vi "my trafic light control.vi"() -> ()   [LabVIEW 2018]
panel:
  in  "stop":bool
  in  "START":bool
  out "Timer 4":u8
  out "Timer 3":u8
  out "Timer 2":u8
  out "Timer":u8
  out "Traffic Light 4":cluster{"Red":bool, "Yellow":bool, "Green":bool}
  out "Traffic Light 3":cluster{"Red":bool, "Yellow":bool, "Green":bool}
  out "Traffic Light 2":cluster{"Red":bool, "Yellow":bool, "Green":bool}
  out "Traffic Light":cluster{"Red":bool, "Yellow":bool, "Green":bool}
  # "GREEN TIME - 10 SECONDS\nRED TIME - \nYELLOW TIME - 2 SECONDS"
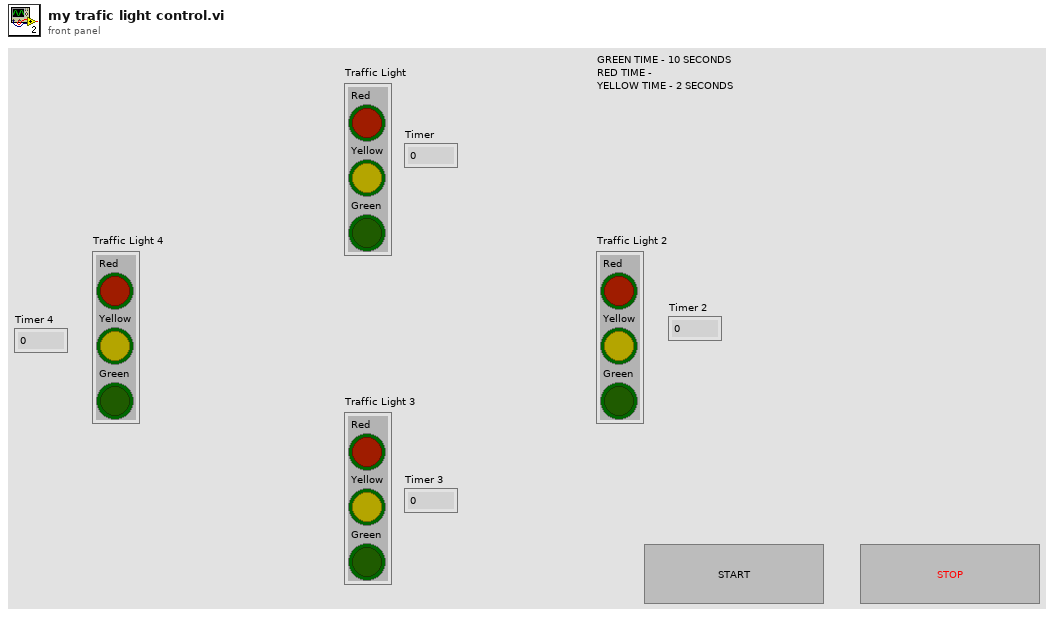
[diagram p1: front panel]
types:
  T1 = enum16{"START", "TL1R", "TL1Y", "TL1G", "TL2R", "TL2Y", "TL2G", "TL3R", "TL3Y", "TL3G", "TL4R", "TL4Y", "TL4G", "STOP"}
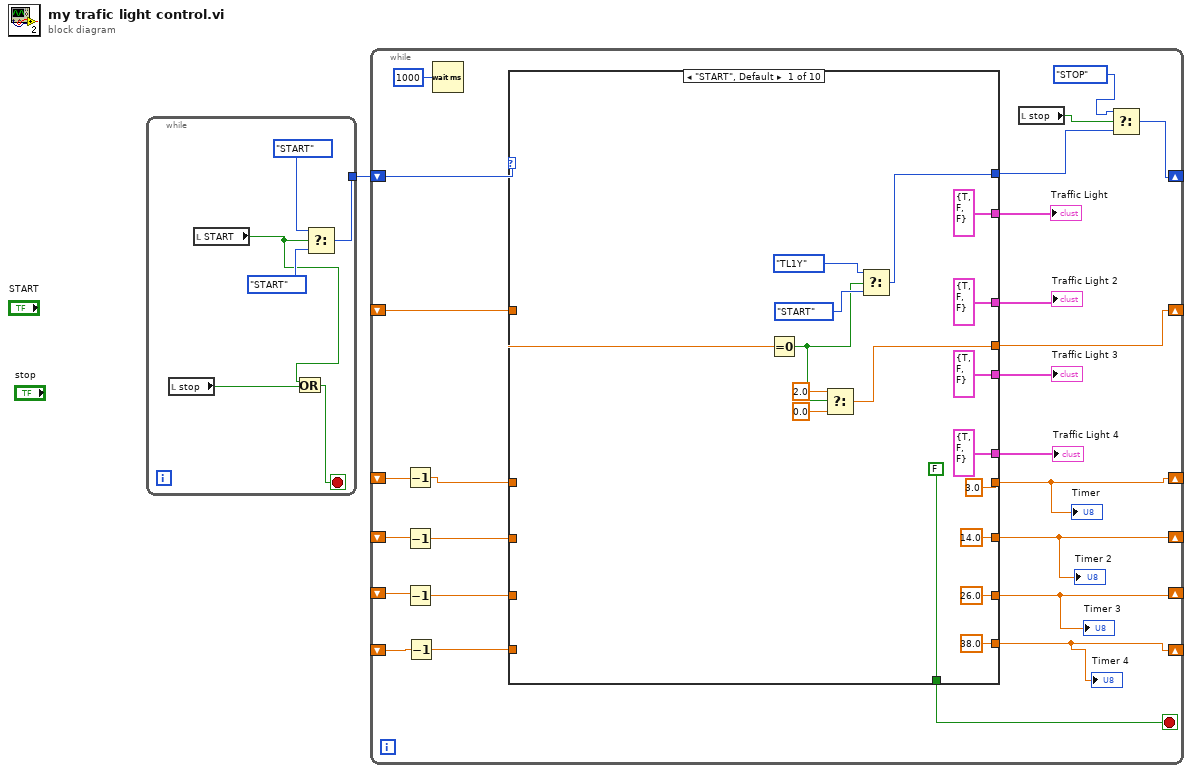
[diagram p0: block diagram]
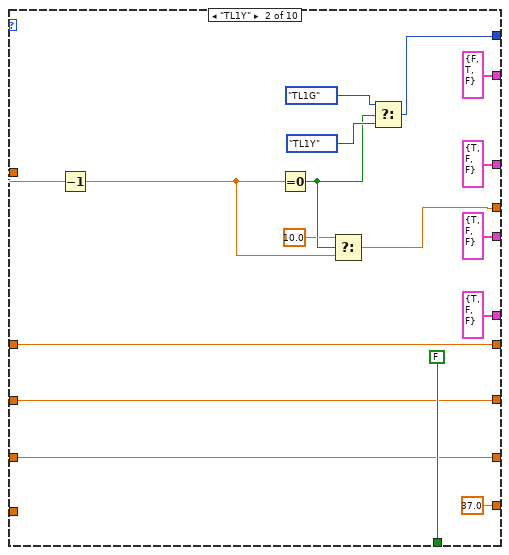
[diagram p2: hidden frame]
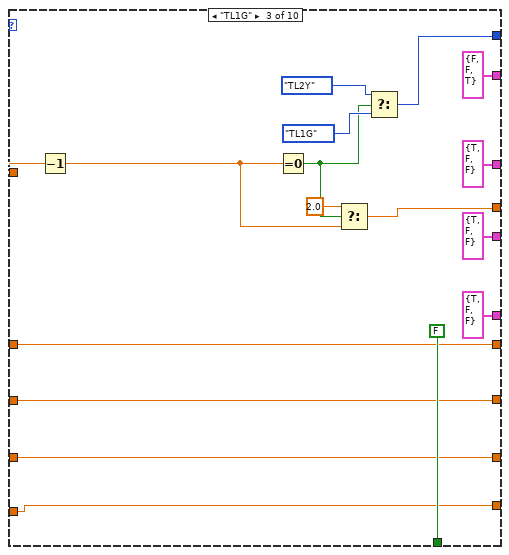
[diagram p3: hidden frame]
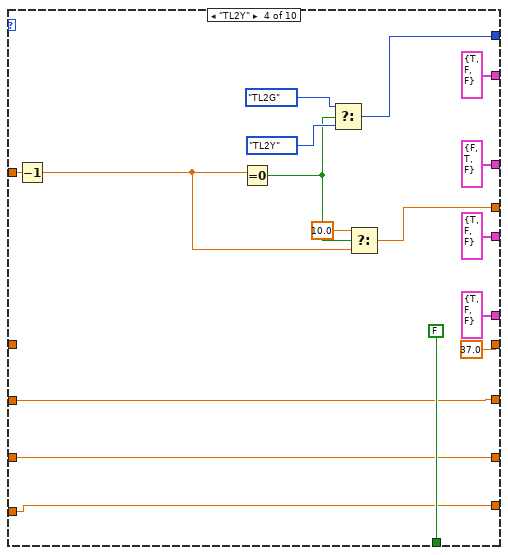
[diagram p4: hidden frame]
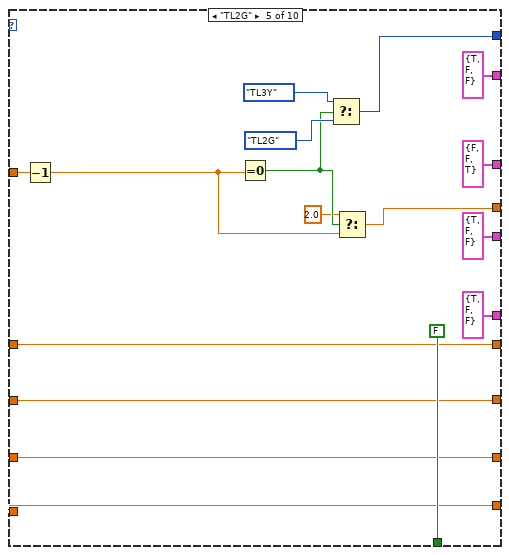
[diagram p5: hidden frame]
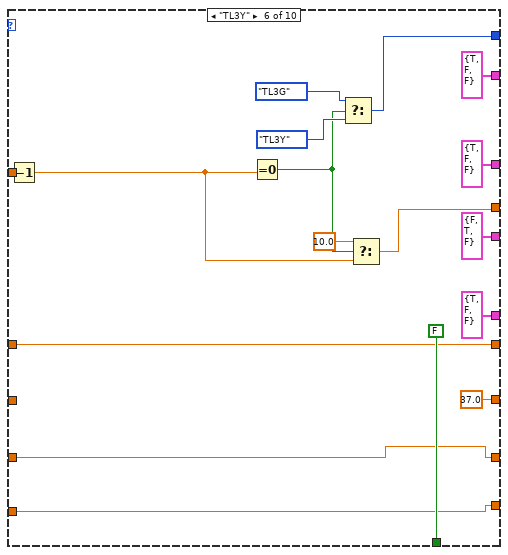
[diagram p6: hidden frame]
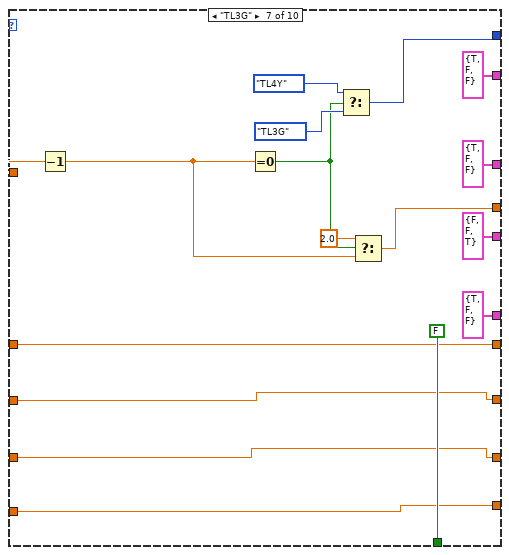
[diagram p7: hidden frame]
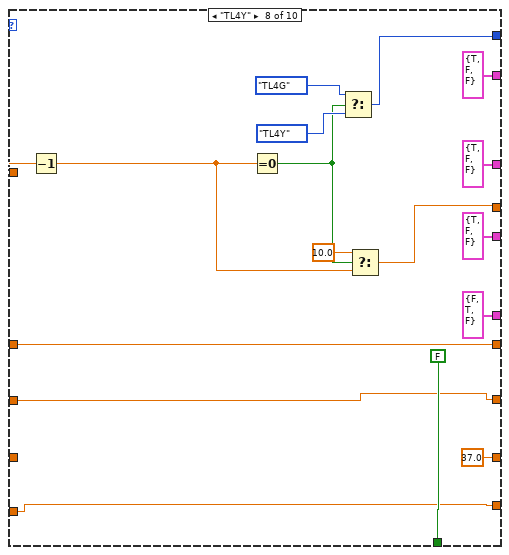
[diagram p8: hidden frame]
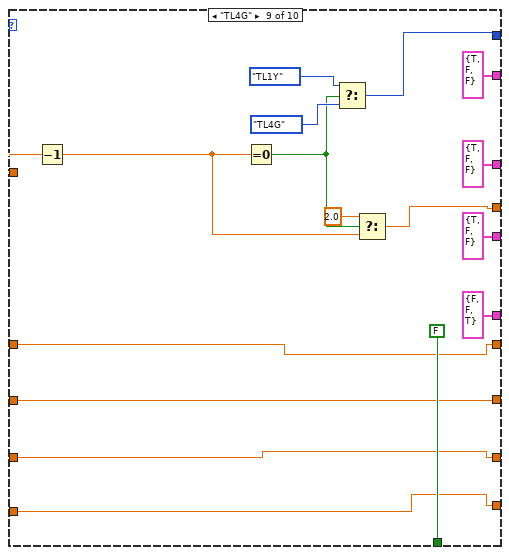
[diagram p9: hidden frame]
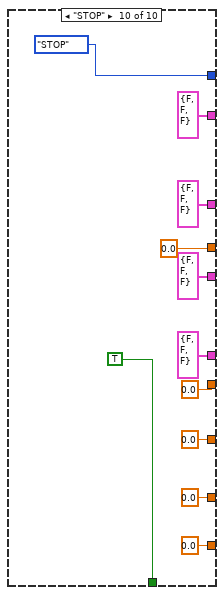
[diagram p10: hidden frame]
diagram:
  n1 = while {
    tunnel: [w7] -> w1
    stop <- w4 stop-if-true
    n2 = local read "stop"() -> (w2:bool)
    n3 = local read "START"() -> (w3:bool)
    n4 = Or(x=w3, y=w2) -> (x .or. y?=w4:bool)
    n5 = Select(t=T1."START", s=w3, f=T1."START") -> (s? t:f=w7:T1)
  }
  n6 = while {
    shift-right: [w10] -> _
    shift-left: w1 -> [w28]
    shift-right: [w25] -> _
    shift-left: _ -> [w26]
    shift-right: [w16] -> _
    shift-left: _ -> [w24]
    shift-right: [w15] -> _
    shift-left: _ -> [w22]
    shift-right: [w14] -> _
    shift-left: _ -> [w19]
    shift-right: [w13] -> _
    shift-left: _ -> [w18]
    stop <- w12 stop-if-true
    n7 = Decrement(x=w24) -> (x-1=w23:dbl)
    n8 = Decrement(x=w22) -> (x-1=w21:dbl)
    n9 = Decrement(x=w19) -> (x-1=w20:dbl)
    n10 = Decrement(x=w18) -> (x-1=w17:dbl)
    n11 = Wait (ms)(milliseconds to wait=u32 1000) -> ()  [unwired: 1 out]
    n12 = case shown="\"START\", Default" w28 {
      tunnel: [cluster{"Red":bool, "Yellow":bool, "Green":bool} {"Red"=TRUE, "Yellow"=FALSE, "Green"=FALSE} ("Traffic Light 4") cluster{"Red":bool, "Yellow":bool, "Green":bool} {"Red"=TRUE, "Yellow"=FALSE, "Green"=FALSE} ("Traffic Light 4") cluster{"Red":bool, "Yellow":bool, "Green":bool} {"Red"=TRUE, "Yellow"=FALSE, "Green"=FALSE} ("Traffic Light 4") cluster{"Red":bool, "Yellow":bool, "Green":bool} {"Red"=TRUE, "Yellow"=FALSE, "Green"=FALSE} ("Traffic Light 4") cluster{"Red":bool, "Yellow":bool, "Green":bool} {"Red"=TRUE, "Yellow"=FALSE, "Green"=FALSE} ("Traffic Light 4") cluster{"Red":bool, "Yellow":bool, "Green":bool} {"Red"=TRUE, "Yellow"=FALSE, "Green"=FALSE} ("Traffic Light 4") cluster{"Red":bool, "Yellow":bool, "Green":bool} {"Red"=TRUE, "Yellow"=FALSE, "Green"=FALSE} ("Traffic Light 4") cluster{"Red":bool, "Yellow":bool, "Green":bool} {"Red"=FALSE, "Yellow"=TRUE, "Green"=FALSE} ("Traffic Light 4") cluster{"Red":bool, "Yellow":bool, "Green":bool} {"Red"=FALSE, "Yellow"=FALSE, "Green"=TRUE} ("Traffic Light 4") cluster{"Red":bool, "Yellow":bool, "Green":bool} {"Red"=FALSE, "Yellow"=FALSE, "Green"=FALSE} ("Traffic Light 4")] -> w32
      tunnel: [cluster{"Red":bool, "Yellow":bool, "Green":bool} {"Red"=TRUE, "Yellow"=FALSE, "Green"=FALSE} ("Traffic Light 3") cluster{"Red":bool, "Yellow":bool, "Green":bool} {"Red"=TRUE, "Yellow"=FALSE, "Green"=FALSE} ("Traffic Light 3") cluster{"Red":bool, "Yellow":bool, "Green":bool} {"Red"=TRUE, "Yellow"=FALSE, "Green"=FALSE} ("Traffic Light 3") cluster{"Red":bool, "Yellow":bool, "Green":bool} {"Red"=TRUE, "Yellow"=FALSE, "Green"=FALSE} ("Traffic Light 3") cluster{"Red":bool, "Yellow":bool, "Green":bool} {"Red"=TRUE, "Yellow"=FALSE, "Green"=FALSE} ("Traffic Light 3") cluster{"Red":bool, "Yellow":bool, "Green":bool} {"Red"=FALSE, "Yellow"=TRUE, "Green"=FALSE} ("Traffic Light 3") cluster{"Red":bool, "Yellow":bool, "Green":bool} {"Red"=FALSE, "Yellow"=FALSE, "Green"=TRUE} ("Traffic Light 3") cluster{"Red":bool, "Yellow":bool, "Green":bool} {"Red"=TRUE, "Yellow"=FALSE, "Green"=FALSE} ("Traffic Light 3") cluster{"Red":bool, "Yellow":bool, "Green":bool} {"Red"=TRUE, "Yellow"=FALSE, "Green"=FALSE} ("Traffic Light 3") cluster{"Red":bool, "Yellow":bool, "Green":bool} {"Red"=FALSE, "Yellow"=FALSE, "Green"=FALSE} ("Traffic Light 3")] -> w31
      tunnel: [cluster{"Red":bool, "Yellow":bool, "Green":bool} {"Red"=TRUE, "Yellow"=FALSE, "Green"=FALSE} ("Traffic Light 2") cluster{"Red":bool, "Yellow":bool, "Green":bool} {"Red"=TRUE, "Yellow"=FALSE, "Green"=FALSE} ("Traffic Light 2") cluster{"Red":bool, "Yellow":bool, "Green":bool} {"Red"=TRUE, "Yellow"=FALSE, "Green"=FALSE} ("Traffic Light 2") cluster{"Red":bool, "Yellow":bool, "Green":bool} {"Red"=FALSE, "Yellow"=TRUE, "Green"=FALSE} ("Traffic Light 2") cluster{"Red":bool, "Yellow":bool, "Green":bool} {"Red"=FALSE, "Yellow"=FALSE, "Green"=TRUE} ("Traffic Light 2") cluster{"Red":bool, "Yellow":bool, "Green":bool} {"Red"=TRUE, "Yellow"=FALSE, "Green"=FALSE} ("Traffic Light 2") cluster{"Red":bool, "Yellow":bool, "Green":bool} {"Red"=TRUE, "Yellow"=FALSE, "Green"=FALSE} ("Traffic Light 2") cluster{"Red":bool, "Yellow":bool, "Green":bool} {"Red"=TRUE, "Yellow"=FALSE, "Green"=FALSE} ("Traffic Light 2") cluster{"Red":bool, "Yellow":bool, "Green":bool} {"Red"=TRUE, "Yellow"=FALSE, "Green"=FALSE} ("Traffic Light 2") cluster{"Red":bool, "Yellow":bool, "Green":bool} {"Red"=FALSE, "Yellow"=FALSE, "Green"=FALSE} ("Traffic Light 2")] -> w30
      tunnel: [cluster{"Red":bool, "Yellow":bool, "Green":bool} {"Red"=TRUE, "Yellow"=FALSE, "Green"=FALSE} ("Traffic Light") cluster{"Red":bool, "Yellow":bool, "Green":bool} {"Red"=FALSE, "Yellow"=TRUE, "Green"=FALSE} ("Traffic Light") cluster{"Red":bool, "Yellow":bool, "Green":bool} {"Red"=FALSE, "Yellow"=FALSE, "Green"=TRUE} ("Traffic Light") cluster{"Red":bool, "Yellow":bool, "Green":bool} {"Red"=TRUE, "Yellow"=FALSE, "Green"=FALSE} ("Traffic Light") cluster{"Red":bool, "Yellow":bool, "Green":bool} {"Red"=TRUE, "Yellow"=FALSE, "Green"=FALSE} ("Traffic Light") cluster{"Red":bool, "Yellow":bool, "Green":bool} {"Red"=TRUE, "Yellow"=FALSE, "Green"=FALSE} ("Traffic Light") cluster{"Red":bool, "Yellow":bool, "Green":bool} {"Red"=TRUE, "Yellow"=FALSE, "Green"=FALSE} ("Traffic Light") cluster{"Red":bool, "Yellow":bool, "Green":bool} {"Red"=TRUE, "Yellow"=FALSE, "Green"=FALSE} ("Traffic Light") cluster{"Red":bool, "Yellow":bool, "Green":bool} {"Red"=TRUE, "Yellow"=FALSE, "Green"=FALSE} ("Traffic Light") cluster{"Red":bool, "Yellow":bool, "Green":bool} {"Red"=FALSE, "Yellow"=FALSE, "Green"=FALSE} ("Traffic Light")] -> w29
      tunnel: [w43 w60 w77 w94 w111 w128 w145 w162 w179 T1."STOP"] -> w9
      tunnel: w26 -> [w40 w59 w76 w92 w110 w127 w144 w161 w178 _]
      tunnel: [w41 w53 w69 w90 w108 w124 w141 w159 w176 0.0 ("t")] -> w25
      tunnel: [FALSE FALSE FALSE FALSE FALSE FALSE FALSE FALSE FALSE TRUE] -> w12
      tunnel: [3.0 w50 w67 37.0 w101 w121 w138 w155 w172 0.0] -> w16
      tunnel: [14.0 w55 w72 w87 w104 37.0 w137 w154 w171 0.0] -> w15
      tunnel: [26.0 w54 w71 w86 w103 w120 w136 37.0 w170 0.0] -> w14
      tunnel: w23 -> [_ w50 w67 _ w101 w121 w138 w155 w172 _]
      tunnel: w21 -> [_ w55 w72 w87 w104 _ w137 w154 w171 _]
      tunnel: w20 -> [_ w54 w71 w86 w103 w120 w136 _ w170 _]
      tunnel: w17 -> [_ _ w70 w85 w102 w119 w135 w153 w169 _]
      tunnel: [38.0 37.0 w70 w85 w102 w119 w135 w153 w169 0.0] -> w13
      frame "START", Default {
        n13 = Equal To 0?(x=w40) -> (x = 0?=w42:bool)
        n14 = Select(t=2.0, s=w42, f=0.0) -> (s? t:f=w41:dbl)
        n15 = Select(t=T1."TL1Y", s=w42, f=T1."START") -> (s? t:f=w43:T1)
      }
      frame "TL1Y" {
        n16 = Decrement(x=w59) -> (x-1=w52:dbl)
        n17 = Equal To 0?(x=w52) -> (x = 0?=w58:bool)
        n18 = Select(t=10.0, s=w58, f=w52) -> (s? t:f=w53:dbl)
        n19 = Select(t=T1."TL1G", s=w58, f=T1."TL1Y") -> (s? t:f=w60:T1)
      }
      frame "TL1G" {
        n20 = Decrement(x=w76) -> (x-1=w68:dbl)
        n21 = Equal To 0?(x=w68) -> (x = 0?=w75:bool)
        n22 = Select(t=2.0, s=w75, f=w68) -> (s? t:f=w69:dbl)
        n23 = Select(t=T1."TL2Y", s=w75, f=T1."TL1G") -> (s? t:f=w77:T1)
      }
      frame "TL2Y" {
        n24 = Decrement(x=w92) -> (x-1=w88:dbl)
        n25 = Equal To 0?(x=w88) -> (x = 0?=w93:bool)
        n26 = Select(t=T1."TL2G", s=w93, f=T1."TL2Y") -> (s? t:f=w94:T1)
        n27 = Select(t=10.0, s=w93, f=w88) -> (s? t:f=w90:dbl)
      }
      frame "TL2G" {
        n28 = Decrement(x=w110) -> (x-1=w105:dbl)
        n29 = Equal To 0?(x=w105) -> (x = 0?=w109:bool)
        n30 = Select(t=T1."TL3Y", s=w109, f=T1."TL2G") -> (s? t:f=w111:T1)
        n31 = Select(t=2.0, s=w109, f=w105) -> (s? t:f=w108:dbl)
      }
      frame "TL3Y" {
        n32 = Decrement(x=w127) -> (x-1=w122:dbl)
        n33 = Equal To 0?(x=w122) -> (x = 0?=w126:bool)
        n34 = Select(t=T1."TL3G", s=w126, f=T1."TL3Y") -> (s? t:f=w128:T1)
        n35 = Select(t=10.0, s=w126, f=w122) -> (s? t:f=w124:dbl)
      }
      frame "TL3G" {
        n36 = Decrement(x=w144) -> (x-1=w139:dbl)
        n37 = Equal To 0?(x=w139) -> (x = 0?=w143:bool)
        n38 = Select(t=T1."TL4Y", s=w143, f=T1."TL3G") -> (s? t:f=w145:T1)
        n39 = Select(t=2.0, s=w143, f=w139) -> (s? t:f=w141:dbl)
      }
      frame "TL4Y" {
        n40 = Decrement(x=w161) -> (x-1=w156:dbl)
        n41 = Equal To 0?(x=w156) -> (x = 0?=w160:bool)
        n42 = Select(t=T1."TL4G", s=w160, f=T1."TL4Y") -> (s? t:f=w162:T1)
        n43 = Select(t=10.0, s=w160, f=w156) -> (s? t:f=w159:dbl)
      }
      frame "TL4G" {
        n44 = Decrement(x=w178) -> (x-1=w173:dbl)
        n45 = Equal To 0?(x=w173) -> (x = 0?=w177:bool)
        n46 = Select(t=T1."TL1Y", s=w177, f=T1."TL4G") -> (s? t:f=w179:T1)
        n47 = Select(t=2.0, s=w177, f=w173) -> (s? t:f=w176:dbl)
      }
      frame "STOP" {
      }
    }
    "Traffic Light" <- w29
    "Traffic Light 2" <- w30
    "Traffic Light 3" <- w31
    "Traffic Light 4" <- w32
    "Timer" <- w16
    "Timer 2" <- w15
    "Timer 3" <- w14
    "Timer 4" <- w13
    n48 = local read "stop"() -> (w8:bool)
    n49 = Select(t=T1."STOP", s=w8, f=w9) -> (s? t:f=w10:T1)
  }
